vi "read default menu name.vi"(8 "error in":errorcluster, 11 "Engine Parent Editor Node in":refnum<class "Engine Parent Editor Node.lvclass">) -> (0 "error out":errorcluster, 2 "default menu name":string, 3 "Engine Parent Editor Node out":refnum<class "Engine Parent Editor Node.lvclass">)   [LabVIEW 2013, in "PL Framework Configuration Tool.lvlib" / "Engine Parent Editor Node.lvclass"]
uses:
  Engine Parent Editor Node.lvclass
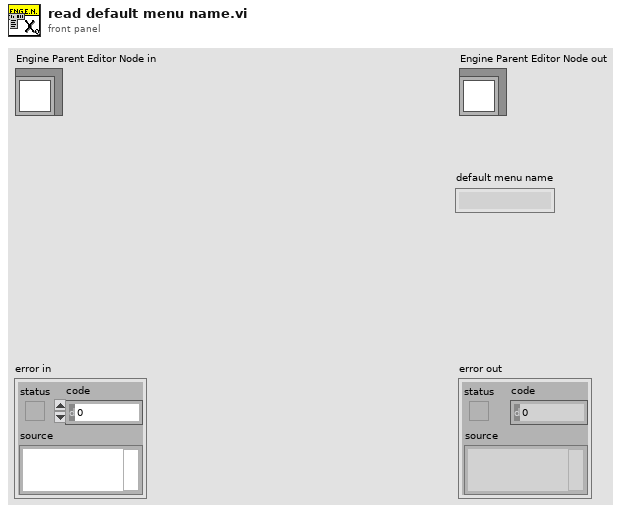
[diagram p1: front panel]
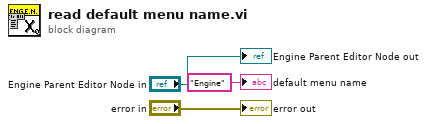
[diagram p0: block diagram]
diagram:
  "error out" <- "error in"
  "Engine Parent Editor Node out" <- "Engine Parent Editor Node in"
  "default menu name" <- "Engine" ("default menu name")
